vi "Save Settings to XML.vi"(8 "error in (no error)":errorcluster, 11 "Settings":T1={"Hardware Configuration"={"DAQmx Channel"="", "Max Input"=0.0, "Min Input"=0.0, "Sample Rate"=0.0, "DAQmx Task"=""}, "Logging Configuration"={"Log File Base Path"=path "", "TDMS File Reference"=refnum, "Samples to Save"=0, "Trigger - Time"=0, "Trigger - Threshold"=0.0, "Trigger - Channel"=0, "Enable Time Trigger"=FALSE, "Enable Threshold Trigger"=FALSE, "Always Log"=FALSE}, "MSpeed AO HW Config"={"MSpeed AO Channel"="", "Sample Rate(Hz)"=1000.0, "MSpeed AO Task"=""}, "Motor Config"={"VISA resource name"="", "Speed and Duration"=[]}, "2P Trigger Config"={"DO Line"="Dev1/port0/line0"}} {"Motor Config"."Speed and Duration"."Duration (sec)" min=0.0 max=100.0 step=0.1 format="%.1f"; "Motor Config"."Speed and Duration"."Speed (%)" min=0 max=100 step=1 format="%.1f"}) -> (0 "error out":errorcluster)   [LabVIEW 2016, in "Settings.lvlib"]
doc: "Saves the \"User Specified\" configuration data to an XML file. This is used to remember the users settings between executions."
uses:
  Settings.lvlib
  Settings.ctl
  Acquisition/Hardware Configuration.ctl
  Logging/Logging Configuration.ctl
  Motor Speed/MSpeed AO HW Config.ctl
  Motor Control/Motor Control Config.ctl
  Motor Control/Speed and Duration.ctl
  2P Trigger/2P Trigger Config.ctl
  <vilib>/Utility/xml.llb/Write to XML File(string).vi
  Acquisition/Acquisition.lvlib
  Logging/Logging.lvlib
  Motor Speed/Motor Speed AO.lvlib
  Motor Control/Motor Control.lvlib
  2P Trigger/2P Trigger.lvlib
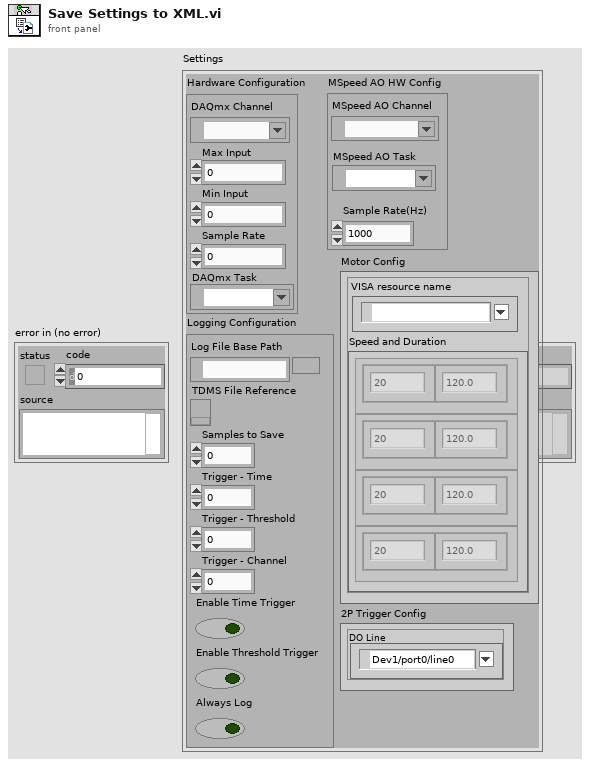
[diagram p1: front panel]
types:
  T1 = typedef "Settings.lvlib/Settings.ctl" = cluster{"Hardware Configuration":T2, "Logging Configuration":T3, "MSpeed AO HW Config":T4, "Motor Config":T5, "2P Trigger Config":T7}
  T2 = typedef "Acquisition.lvlib/Hardware Configuration.ctl" = cluster{"DAQmx Channel":tag, "Max Input":dbl, "Min Input":dbl, "Sample Rate":dbl, "DAQmx Task":refnum<k21>}
  T3 = typedef "Logging.lvlib/Logging Configuration.ctl" = cluster{"Log File Base Path":path, "TDMS File Reference":refnum<k34>, "Samples to Save":u32, "Trigger - Time":u32, "Trigger - Threshold":dbl, "Trigger - Channel":u32, "Enable Time Trigger":bool, "Enable Threshold Trigger":bool, "Always Log":bool}
  T4 = typedef "Motor Speed AO.lvlib/MSpeed AO HW Config.ctl" = cluster{"MSpeed AO Channel":tag, "Sample Rate(Hz)":dbl, "MSpeed AO Task":refnum<k21>}
  T5 = typedef "Motor Control.lvlib/Motor Control Config.ctl" = cluster{"VISA resource name":refnum<visa-resource-name>, "Speed and Duration":T6[]}
  T6 = typedef "Motor Control.lvlib/Speed and Duration.ctl" = cluster{"Speed (%)":i32, "Duration (sec)":dbl}
  T7 = typedef "2P Trigger.lvlib/2P Trigger Config.ctl" = cluster{"DO Line":tag}
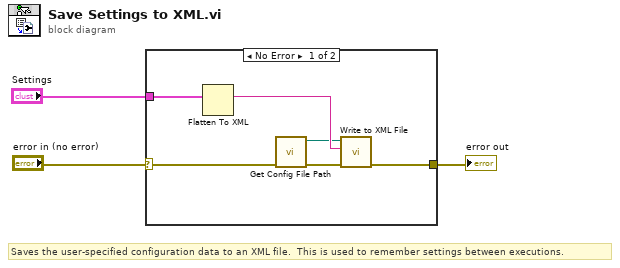
[diagram p0: block diagram]
diagram:
  # "Saves the user-specified configuration data to an XML file.  This is used to remember settings between executions."
  n1 = case shown="No Error" "error in (no error)" {
    selector: "error in (no error)" -> [w5 w10]
    tunnel: [w7 w10] -> w2
    tunnel: "Settings" -> [w9 _]
    frame No Error {
      n2 = Flatten To XML(anything=w9) -> (xml string=w8:string)
      n3 = call "Get Config File Path.vi"("error in (no error)"=w5) -> ("error out"=w4:errorcluster, "XML File Path"=w6:path)  [unwired: 9 in]
      n4 = call-poly <vilib>:"Write to XML File.vi"("error in (no error)"=w4, "XML Input"=w8, "XML File Path"=w6) -> ("error out"=w7:errorcluster)  [unwired: 6 in, 2 out]
    }
    frame Error {
    }
  }
  "error out" <- w2
